vi "TDMS_ReadBetweenCurs.vi"(5 "通道名":string[](array[string])=["Sinc", "Sin"], 7 "组名称输入":string="Sig Group", 8 "错误输入":errorcluster, 9 "Cur2":cluster{"X":dbl, "Y":dbl}, 10 "Cur1":cluster{"X":dbl, "Y":dbl}, 11 "tdms文件":refnum<k34>) -> (0 "错误输出":errorcluster, 1 "读取时间(s)":dbl, 2 "数据输出":dbl[][](array[numeric]), 3 "tdms file out":refnum<k34>)   [LabVIEW 2011]
panel:
  # "读取两游标之间的所有数据点, 统计读取时间."
  # "考虑用post event把数据传出去?"
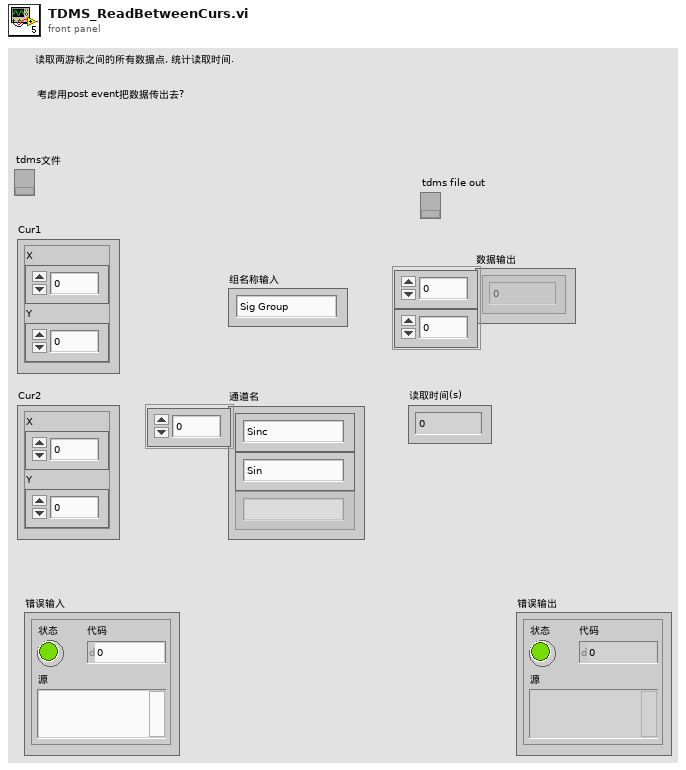
[diagram p1: front panel]
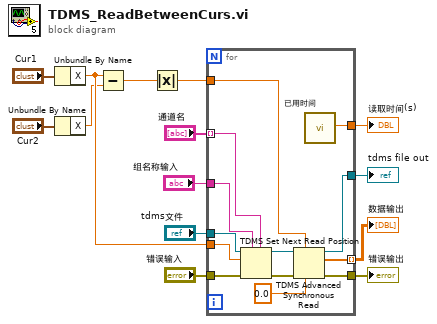
[diagram p0: block diagram]
diagram:
  n1 = Unbundle By Name("Cur1") -> ("X"=w12:dbl)
  n2 = Unbundle By Name("Cur2") -> ("X"=w11:dbl)
  n3 = Subtract(x=w12, y=w11) -> (x-y=w10:dbl)
  n4 = Absolute Value(x=w10) -> (abs(x)=w9:dbl)
  n5 = for {
    tunnel: w12 -> [w26]
    tunnel: w9 -> [w25]
    tunnel: "组名称输入" -> [w23]
    tunnel: "通道名" -> [w22] mode=indexing
    tunnel: [w20] -> w6
    tunnel: "错误输入" -> [w19]
    tunnel: "tdms文件" -> [w18]
    tunnel: [w17] -> w3
    tunnel: [w16] -> w2 mode=indexing
    tunnel: [w15] -> w1
    n6 = TDMS Set Next Read Position(5:w22, 7:w23, 8:w19, 10:w26, 11:w18) -> (0:w21:errorcluster, 3:w27:refnum<k34>)  [unwired: 1 in]
    n7 = TDMS Advanced Synchronous Read(6:0.0, 7:w25, 8:w21, 11:w27) -> (0:w20:errorcluster, 2:w16:dbl[], 3:w17:refnum<k34>)  [unwired: 1 out]
    n8 = call "已用时间"() -> ("Elapsed Time (s)"=w15:dbl)  [unwired: 12 in, 7 out]
  }
  "读取时间(s)" <- w1
  "错误输出" <- w6
  "tdms file out" <- w3
  "数据输出" <- w2
